vi "Debounced Signal.vi"(7 "Reset? (F)":bool, 8 "Debounce Period (5s)":dbl=5.0, 9 "Reset Value":bool, 11 "Signal":bool) -> (0 "Since Last Change (S)":dbl format="%.2f", 3 "Signal (Safe)":bool)   [LabVIEW 2017, in "CSM Shared.lvlib"]
uses:
  CSM Shared.lvlib
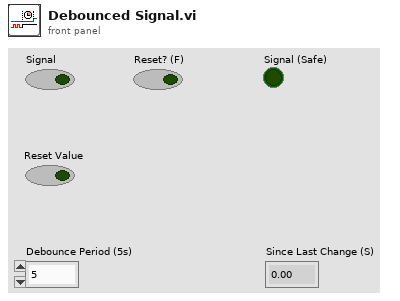
[diagram p1: front panel]
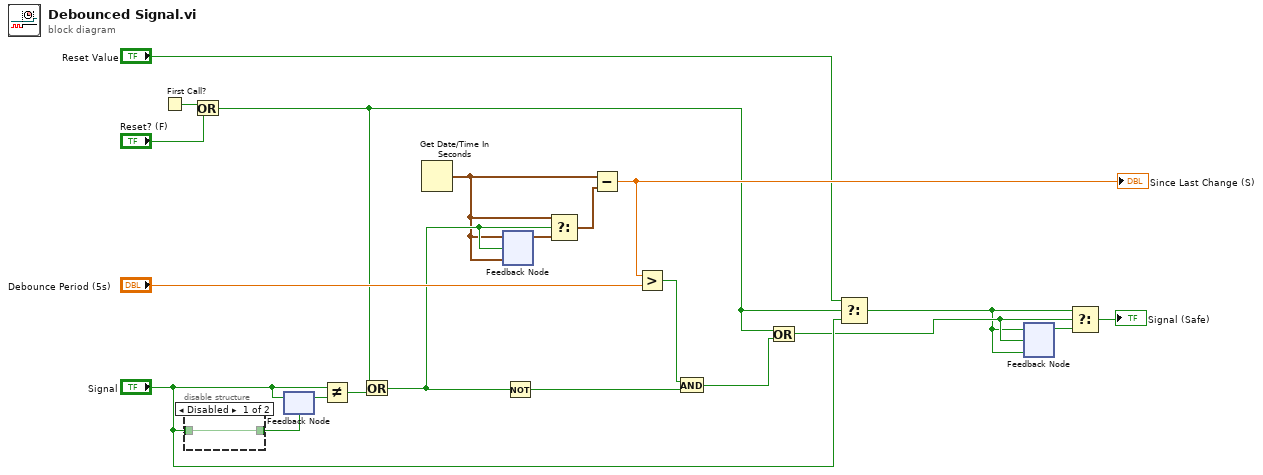
[diagram p0: block diagram]
diagram:
  n1 = First Call?() -> (First Call?: T/F=w21:bool)
  n2 = disable-structure shown="Disabled" {
    disable-tunnel: [w22 _] -> w11
    disable-tunnel: "Signal" -> [w22 _]
    frame Disabled {
    }
    frame Enabled {
    }
  }
  n3 = Or(x=w21, y="Reset? (F)") -> (x .or. y?=w13:bool)
  n4 = feedback #1(w11) -> (w12:bool)
  n5 = feedback-in #1("Signal") -> ()
  n6 = Not Equal?(x="Signal", y=w12) -> (x != y?=w9:bool)
  n7 = Or(x=w13, y=w9) -> (x .or. y?=w7:bool)
  n8 = Get Date/Time In Seconds() -> (seconds since 1Jan1904=w6:timestamp)
  n9 = feedback #2(w6) -> (w8:timestamp)
  n10 = feedback-in #2(w6, w7) -> ()
  n11 = Not(x=w7) -> (.not. x?=w16:bool)
  n12 = Select(t=w6, s=w7, f=w8) -> (s? t:f=w5:timestamp)
  n13 = Subtract(x=w6, y=w5) -> (x-y=w19:dbl)
  "Since Last Change (S)" <- w19
  n14 = Greater?(x=w19, y="Debounce Period (5s)") -> (0:w17:bool)
  n15 = And(x=w17, y=w16) -> (x .and. y?=w15:bool)
  n16 = Or(x=w13, y=w15) -> (x .or. y?=w3:bool)
  n17 = Select(t="Reset Value", s=w13, f="Signal") -> (s? t:f=w2:bool)
  n18 = feedback #3(w2) -> (w4:bool)
  n19 = feedback-in #3(w2, w3) -> ()
  n20 = Select(t=w2, s=w3, f=w4) -> (s? t:f=→"Signal (Safe)":bool)
